vi "ALD valve control.vi"() -> ()   [LabVIEW 2024]
uses:
  <vilib>/MakerHub/LINX/Public/Peripherals/Digital/Digital Write N Chans.vi
  <vilib>/MakerHub/LINX/Private/Local IO/LinxDigitalWrite.vi
  <vilib>/MakerHub/LINX/Public/Utilities/Check Channel.vi
  <vilib>/MakerHub/LINX/Private/Local IO/Handle Errors.vi
  <vilib>/MakerHub/LINX/Public/Utilities/Open Local.vi
  <vilib>/MakerHub/LINX/Private/Utilties/Generate Error.vi
  <vilib>/MakerHub/LINX/LMH-LINX.lvlib
panel:
  out "Current Cycle":dbl
  in  "Oxidizer Purge 2 (s)":dbl
  in  "Oxidizer Pulse 2 (s)":dbl
  out "P2V":bool
  in  "Precursor 2 Purge (s)":dbl
  in  "Precursor 2 Pulse (s)":dbl
  in  "N [every (N+1)th Cycle]":dbl
  out "OV":bool
  out "P1V":bool
  in  "Oxidizer Purge 1 (s)":dbl
  in  "Oxidizer Pulse 1 (s)":dbl
  in  "Precursor 1 Purge (s)":dbl
  in  "Precursor 1 Pulse (s)":dbl
  in  "Number of Cycles":dbl
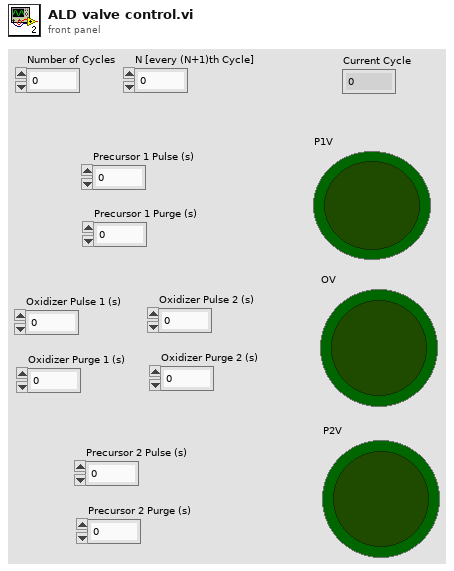
[diagram p1: front panel]
types:
  T1 = typedef "LMH-LINX.lvlib/LINX Ref.ctl" = cluster{"IO":T2, "Interface":T3, "LINX Device Config":T4}
  T2 = typedef "LMH-LINX.lvlib/Platform.ctl" = enum16{"Remote", "Local"}
  T3 = typedef "LMH-LINX.lvlib/Interface.ctl" = enum16{"Serial", "TCP"}
  T4 = typedef "LMH-LINX.lvlib/Device.lvlib/LINX Device Config.ctl" = cluster{"Interface":T3, "COM Port":refnum<visa-resource-name>, "TCP Configuration":T5, "Device Family":u8, "Device ID":u8, "Device Name":string, "TCP Ref":refnum<k5>, "Channels":T6}
  T5 = typedef "LMH-LINX.lvlib/Device.lvlib/TCP Config.ctl" = cluster{"IP Address":string, "Port":u16}
  T6 = typedef "LMH-LINX.lvlib/Channels.ctl" = cluster{"DI":u8[], "DO":u8[], "AI":u8[], "AO":u8[], "PWM":u8[], "QE":u8[], "UART":u8[], "I2C 2":u8[], "SPI":u8[], "CAN":u8[], "Servo":u8[], "AI Ref (V)":dbl, "AI Resolution (Bits)":u8, "AO Ref (V)":dbl, "AO Resolution (Bits)":u8}
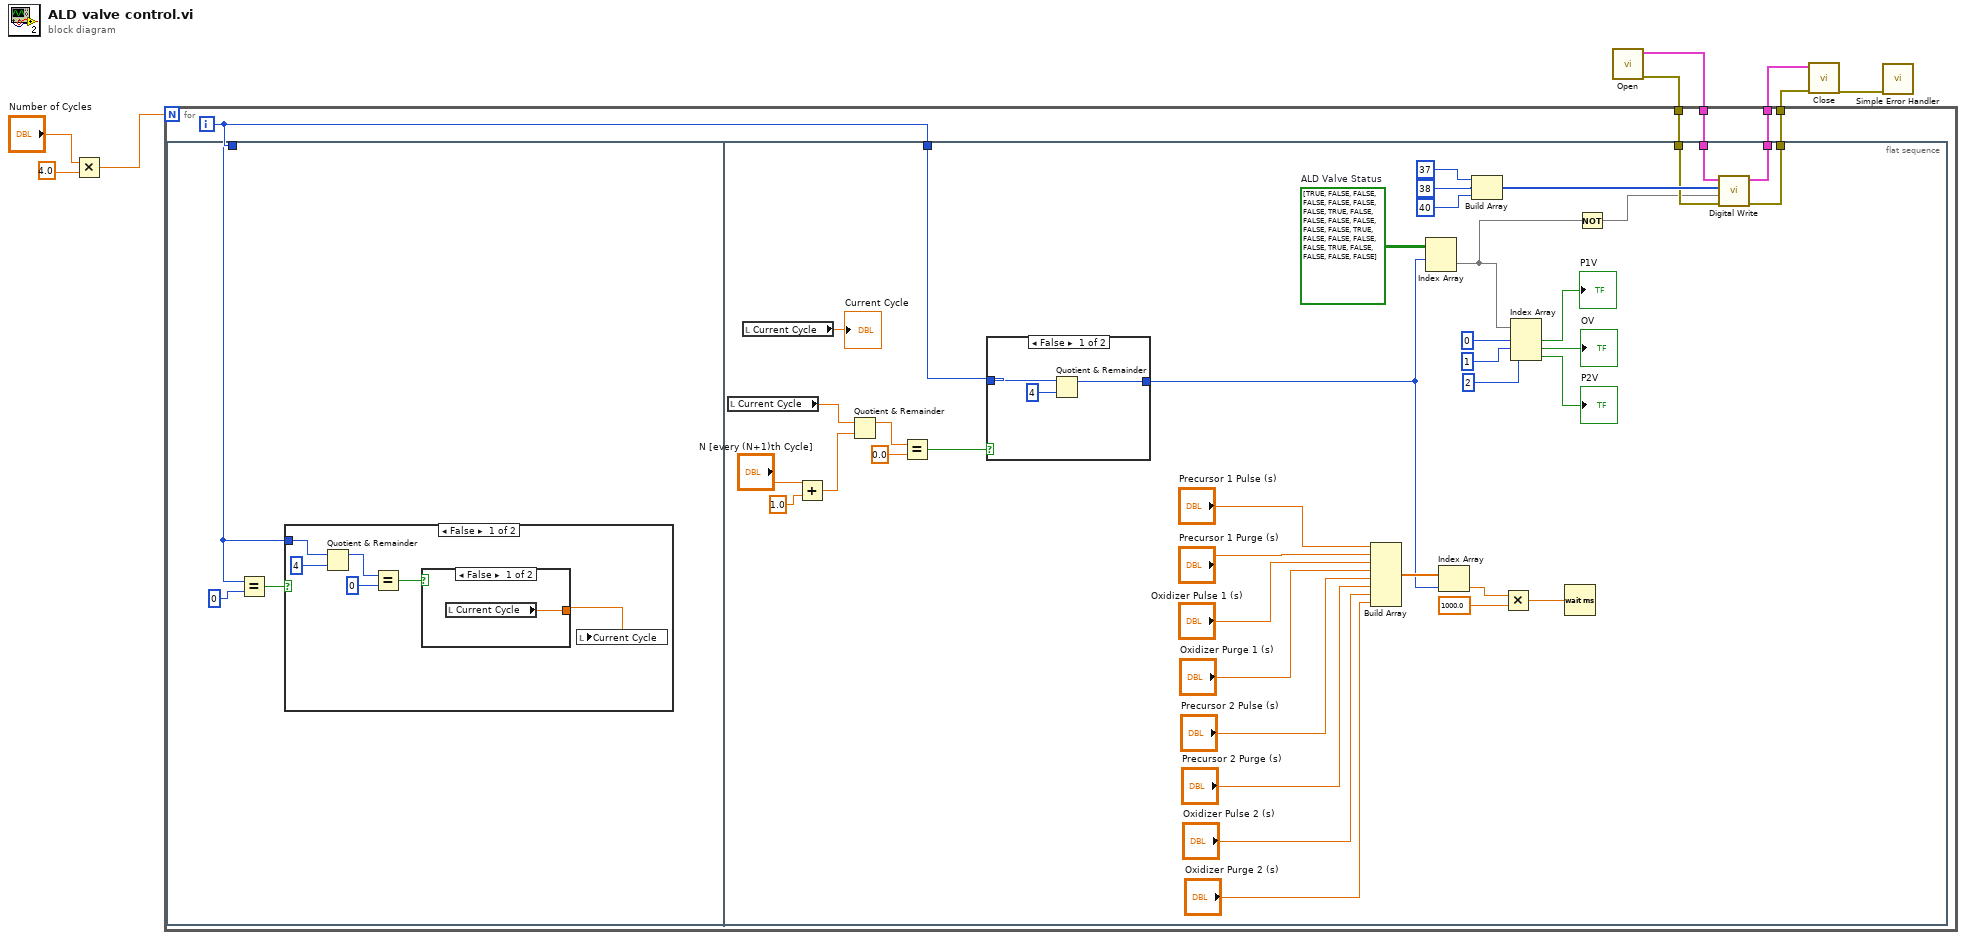
[diagram p0: block diagram]
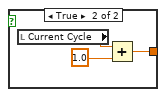
[diagram p2: hidden frame]
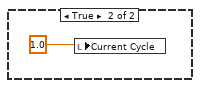
[diagram p3: hidden frame]
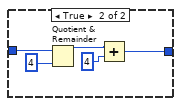
[diagram p4: hidden frame]
diagram:
  n1 = Multiply(x="Number of Cycles", y=4.0) -> (x*y=w8:dbl)
  n2 = call-poly <vilib>:"Open.vi"() -> ("Error Out"=w5:errorcluster, "LINX Resource"=w4:T1)  [unwired: 9 in, 1 out]
  n3 = for {
    N: w8 -> [_]
    tunnel: w5 -> [w12]
    tunnel: w4 -> [w11]
    tunnel: [w10] -> w2
    tunnel: [w9] -> w1
    i -> [w13]
    n4 = flat-sequence {
      tunnel: w13 -> [w14]
      tunnel: w13 -> [w48]
      tunnel: [w34] -> w9
      tunnel: [w33] -> w10
      tunnel: w12 -> [w31]
      tunnel: w11 -> [w30]
      frame #0 {
        n5 = Equal?(x=w14, y=0 ("x")) -> (x = y?=w16:bool)
        n6 = case shown="False" w16 {
          tunnel: w14 -> [w17 _]
          frame False {
            n7 = Quotient & Remainder(x=w17, y=4) -> (x-y*floor(x/y)=w20:i32)  [unwired: 1 out]
            n8 = Equal?(x=w20, y=0) -> (x = y?=w21:bool)
            n9 = case shown="False" w21 {
              tunnel: [w23 w24] -> w22
              frame False {
                n10 = local read "Current Cycle"() -> (w23:dbl)
              }
              frame True {
                n11 = local read "Current Cycle"() -> (w25:dbl)
                n12 = Add(x=w25, y=1.0) -> (x+y=w24:dbl)
              }
            }
            n13 = local write "Current Cycle"(w22) -> ()
          }
          frame True {
            n14 = local write "Current Cycle"(1.0 ("Current Cycle")) -> ()
          }
        }
      }
      frame #1 {
        w42 = bool[][] [[TRUE, FALSE, FALSE], [FALSE, FALSE, FALSE], [FALSE, TRUE, FALSE], [FALSE, FALSE, FALSE], [FALSE, FALSE, TRUE], [FALSE, FALSE, FALSE], [FALSE, TRUE, FALSE], [FALSE, FALSE, FALSE]]  # ALD Valve Status
        n15 = local read "Current Cycle"() -> (w62:dbl)
        n16 = local read "Current Cycle"() -> (→"Current Cycle":dbl)
        n17 = Add(x="N [every (N+1)th Cycle]", y=1.0) -> (x+y=w64:dbl)
        n18 = Quotient & Remainder(x=w62, y=w64) -> (x-y*floor(x/y)=w63:dbl)  [unwired: 1 out]
        n19 = Equal?(x=w63, y=0.0) -> (x = y?=w65:bool)
        n20 = case shown="False" w65 {
          tunnel: w48 -> [w69 w74]
          tunnel: [w67 w70] -> w40
          frame False {
            n21 = Quotient & Remainder(x=w69, y=4) -> (x-y*floor(x/y)=w67:i32)  [unwired: 1 out]
          }
          frame True {
            n22 = Quotient & Remainder(x=w74, y=4) -> (x-y*floor(x/y)=w72:i32)  [unwired: 1 out]
            n23 = Add(x=w72, y=4) -> (x+y=w70:i32)
          }
        }
        n24 = Build Array("Precursor 1 Pulse (s)", "Precursor 1 Purge (s)", "Oxidizer Pulse 1 (s)", "Oxidizer Purge 1 (s)", "Precursor 2 Pulse (s)", "Precursor 2 Purge (s)", "Oxidizer Pulse 2 (s)", "Oxidizer Purge 2 (s)") -> (w53:dbl[])
        n25 = Index Array(array=w42, index (row)=w40) -> (element=w29:bool[])  [unwired: 1 in]
        n26 = Index Array(array=w53, index=w40) -> (element=w54:dbl)
        n27 = Build Array(37, 38, 40) -> (w32:i32[])
        n28 = Multiply(x=w54, y=1000.0) -> (x*y=w55:dbl)
        n29 = Index Array(array=w29, index #1=0, index #2=1, index #3=2 ("index")) -> (element #1=→"P1V":bool, element #2=→"OV":bool, element #3=→"P2V":bool)
        n30 = Wait (ms)(milliseconds to wait=w55) -> ()  [unwired: 1 out]
        n31 = Not(x=w29) -> (.not. x?=w28:bool[])
        n32 = call-poly <vilib>:"Digital Write.vi"("Error In"=w31, "Values"=w28, "DO Channels"=w32, "LINX Resource"=w30) -> ("Error Out"=w33:errorcluster, "LINX Resource"=w34:T1)  [unwired: 6 in]
      }
    }
  }
  n33 = call <vilib>:"Close.vi"("Error In"=w2, "LINX Resource"=w1) -> ("Error Out"=w3:errorcluster)  [unwired: 9 in]
  n34 = call <vilib>:"Simple Error Handler.vi"("error in (no error)"=w3) -> ()  [unwired: 4 in, 5 out]
